vi "Conclude.vi"(8 "error in (no error)":errorcluster, 10 "Iterator Settings":T1={"Prepare timeout (ms)"=200, "Iterate timeout (ms)"=50, "Conclude timeout (ms)"=200, "Iterate period (ms)"=200, "Number of iterations"=5, "Time before stop (ms)"=5, "Active Stop Conditions"={"Number of Iterations"=FALSE, "Time Elapsed"=FALSE, "Iteration Result"=FALSE}, "Prepare Msg"=refnum, "Iterate Msg"=refnum, "Conclude Msg"=refnum, "Iterations End Report"=refnum, "Message Priority (Normal)"=enum."Normal"}, 11 "Iterator Actor in":refnum<class "Iterator NR Actor.lvclass">) -> (0 "error out":errorcluster, 3 "Iterator Actor out":refnum<class "Iterator NR Actor.lvclass">)   [LabVIEW 2023, in "Iterator Actor.lvlib" / "Iterator NR Actor.lvclass"]
doc: "Calls the Conclude method of the Client."
uses:
  Iterator NR Actor.lvclass
  Abstract Iterator Actor/Iterator Settings.ctl
  Abstract Iterator Actor Messages/Iterator Report Iterations End Msg/Iterator Report Iterations End Msg.lvclass
  <vilib>/ActorFramework/Message/Message.lvclass
  Abstract Iterator Actor/Active Stop Conditions.ctl
  <vilib>/ActorFramework/Message Enqueuer/Message Priority.ctl
  <vilib>/ActorFramework/Actor/Actor.lvclass/Actor.ctl
  Iterator NR Actor.lvclass/Iterator NR Actor.ctl
  <vilib>/ActorFramework/Batch Msg/Batch Msg.lvclass/Batch Msg.ctl
  <vilib>/ActorFramework/Message Enqueuer/Message Enqueuer.lvclass/Message Enqueuer.ctl
  <vilib>/ActorFramework/Actor/Read Caller Enqueuer.vi
  <vilib>/ActorFramework/Batch Msg/Send Batch.vi
  <vilib>/ActorFramework/Message Enqueuer/Enqueue.vi
  Iterator NR Actor Messages/Request Iteration Notification Msg/Request Iteration Notification Msg.lvclass
  <vilib>/ActorFramework/Batch Msg/Batch Msg.lvclass
  <userlib>/_OpenG.lib/lvdata/lvdata.llb/LVOOP Is Same Or Descendant Class__ogtk.vi
  Abstract Iterator Actor/Read Settings.vi
  <vilib>/ActorFramework/Message Priority Queue/Priority Enqueue.vi
  <vilib>/Utility/error.llb/Error Cluster From Error Code.vi
  Iterator NR Actor Messages/Abstract Iteration Msg/Abstract Iteration Msg.lvclass
  <vilib>/ErrorRing/Error Ring.xnode
  Abstract Iterator Actor/Abstract Iterator Actor.lvclass
  <vilib>/ActorFramework/Message Enqueuer/Message Enqueuer.lvclass
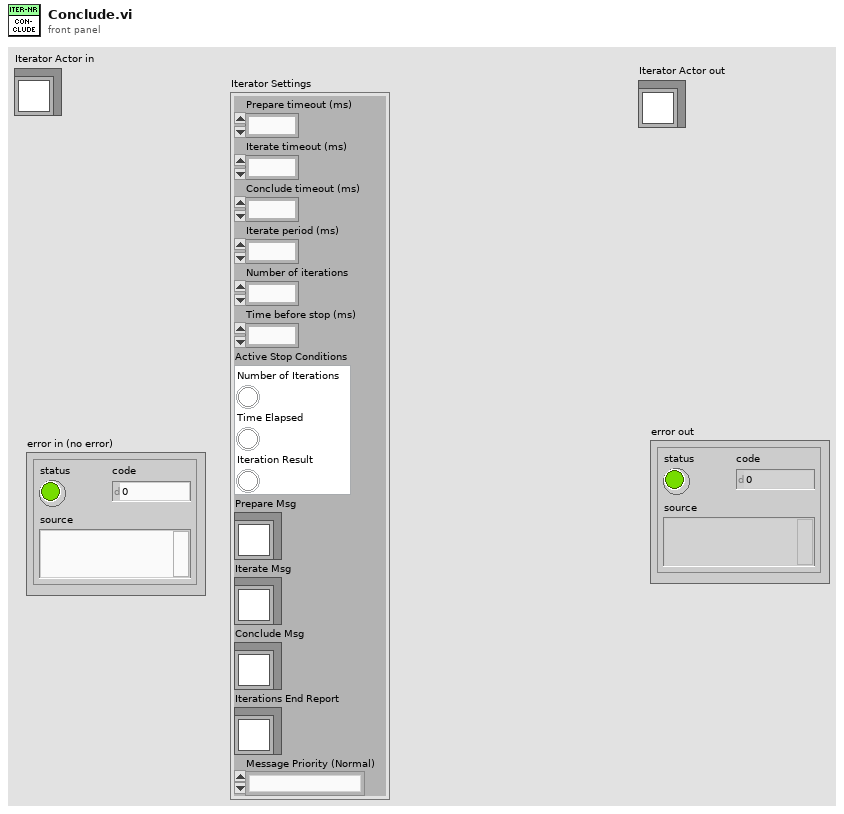
[diagram p1: front panel]
types:
  T1 = typedef "Iterator Actor.lvlib/Abstract Iterator Actor.lvclass/Iterator Settings.ctl" = cluster{"Prepare timeout (ms)":i32, "Iterate timeout (ms)":i32, "Conclude timeout (ms)":i32, "Iterate period (ms)":i32, "Number of iterations":i32, "Time before stop (ms)":i32, "Active Stop Conditions":T2, "Prepare Msg":refnum<class "Message.lvclass">, "Iterate Msg":refnum<class "Message.lvclass">, "Conclude Msg":refnum<class "Message.lvclass">, "Iterations End Report":refnum<class "Iterator Report Iterations End Msg.lvclass">, "Message Priority (Normal)":T3}
  T2 = typedef "Iterator Actor.lvlib/Abstract Iterator Actor.lvclass/Active Stop Conditions.ctl" = cluster{"Number of Iterations":bool, "Time Elapsed":bool, "Iteration Result":bool}
  T3 = typedef "Actor Framework.lvlib/Message Enqueuer.lvclass/Message Priority.ctl" = enum16{"Low", "Normal", "High"}
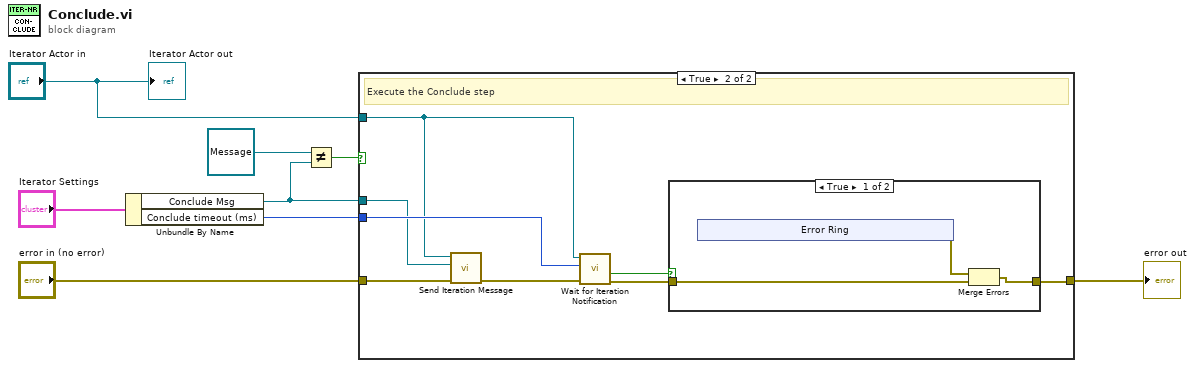
[diagram p0: block diagram]
diagram:
  n1 = Unbundle By Name("Iterator Settings") -> ("Conclude Msg"=w4:refnum<class "Message.lvclass">, "Conclude timeout (ms)"=w8:i32)
  n2 = Not Equal?(x=refnum<class "Message.lvclass"> refnum ("Message"), y=w4) -> (x != y?=w3:bool)
  n3 = case shown="True" w3 {
    tunnel: w8 -> [_ w17]
    tunnel: w4 -> [_ w13]
    tunnel: "error in (no error)" -> [w9 w16]
    tunnel: [w9 w11] -> w5
    tunnel: "Iterator Actor in" -> [_ w14]
    frame False {
      # "Caller did not configure the Conclude step.\nSkip it and go to finish."
    }
    frame True {
      # "Execute the Conclude step"
      n4 = call "Send Iteration Message.vi"("error in (no error)"=w16, "Iteration Msg"=w13, "Iterator NR Actor in"=w14) -> ("error out"=w15:errorcluster)  [unwired: 8 in]
      n5 = call "Wait for Iteration Notification.vi"("error in (no error)"=w15, "timeout in ms (-1)"=w17, "Iterator NR Actor in"=w14) -> ("error out"=w12:errorcluster, "timed out?"=w10:bool)  [unwired: 5 in, 2 out]
      n6 = case shown="True" w10 {
        tunnel: w12 -> [w20 w25]
        tunnel: [w19 w25] -> w11
        frame True {
          n7 = xnode "Error Ring"() -> ("error out"=w18:errorcluster)
          n8 = Merge Errors(w18, w20) -> (w19:errorcluster)
        }
        frame False {
        }
      }
    }
  }
  "error out" <- w5
  "Iterator Actor out" <- "Iterator Actor in"
